vi "IMAQ_Attribute2Control_Enum.vi"(3 "error in (no error)":errorcluster, 4 "IMAQ Attribute":variant, 5 "Refnum (Enum)":refnum<vi>) -> (0 "error out":errorcluster, 1 "dup IMAQ Attribute":variant)   [LabVIEW 2012, in "HGF_VisionTools.lvlib"]
doc: "This Polymorphic VI set IMAQ control properties of type enumeration according to variant inputp value and its attribute."
uses:
  HGF_VisionTools.lvlib
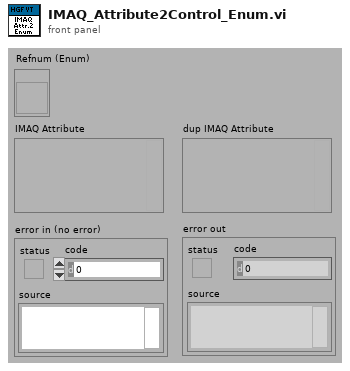
[diagram p1: front panel]
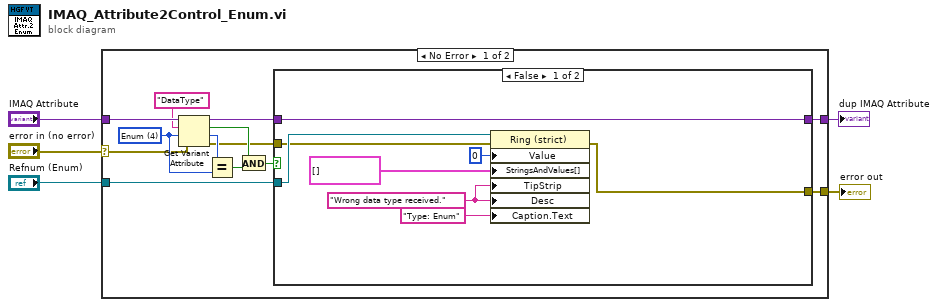
[diagram p0: block diagram]
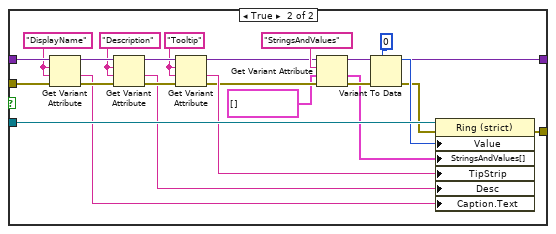
[diagram p2: hidden frame]
diagram:
  n1 = case shown="No Error" "error in (no error)" {
    selector: "error in (no error)" -> [w11 w52]
    tunnel: "IMAQ Attribute" -> [w18 w51]
    tunnel: "Refnum (Enum)" -> [w8 _]
    tunnel: [w7 w52] -> w2
    tunnel: [w6 w51] -> w1
    frame No Error {
      w15 = u32 4 items=["U32", "I64", "DBL", "String", "Enum", "Bool", "Command"] ("Type")
      n2 = Get Variant Attribute(Variant=w18, name="DataType", default value (empty Variant)=w15, error in=w11) -> (duplicate Variant=w10:variant, found=w14:bool, value=w16:u32, error out=w9:errorcluster)
      n3 = Equal?(x=w16, y=w15) -> (x = y?=w13:bool)
      n4 = And(x=w14, y=w13) -> (x .and. y?=w12:bool)
      n5 = case shown="False" w12 {
        tunnel: w10 -> [w26 w50]
        tunnel: w9 -> [w24 w49]
        tunnel: w8 -> [w25 w48]
        tunnel: [w20 w33] -> w7
        tunnel: [w26 w32] -> w6
        frame False {
          w21 = "Wrong data type received." ("Caption.Text")
          n6 = property class="Ring (strict)"(reference=w25, error in=w24, "Value"=u16 0, "StringsAndValues[]"=cluster{"String":string, "Value":u32}[] [] ("Strings And Values []"), "TipStrip"=w21, "Desc"=w21, "Caption.Text"="Type: Enum") -> (error out=w20:errorcluster)  [unwired: 1 out]
        }
        frame True {
          w38 = "Tooltip" ("name")
          w37 = "Description" ("name")
          w36 = "DisplayName" ("name")
          n7 = Get Variant Attribute(Variant=w50, name=w36, default value (empty Variant)=w36, error in=w49) -> (duplicate Variant=w45:variant, value=w34:string, error out=w46:errorcluster)  [unwired: 1 out]
          n8 = Get Variant Attribute(Variant=w45, name=w37, default value (empty Variant)=w37, error in=w46) -> (duplicate Variant=w44:variant, value=w35:string, error out=w47:errorcluster)  [unwired: 1 out]
          n9 = Get Variant Attribute(Variant=w44, name=w38, default value (empty Variant)=w38, error in=w47) -> (duplicate Variant=w31:variant, value=w39:string, error out=w30:errorcluster)  [unwired: 1 out]
          n10 = Get Variant Attribute(Variant=w31, name="StringsAndValues", default value (empty Variant)=cluster{"String":string, "Value":u32}[] [] ("Strings And Values []"), error in=w30) -> (duplicate Variant=w32:variant, value=w27:cluster{"String":string, "Value":u32}[], error out=w42:errorcluster)  [unwired: 1 out]
          n11 = Variant To Data(error in=w42, type=u32 0 ("Value"), Variant=w32) -> (data=w41:u32, error out=w40:errorcluster)
          n12 = property class="Ring (strict)"(reference=w48, error in=w40, "Value"=w41, "StringsAndValues[]"=w27, "TipStrip"=w39, "Desc"=w35, "Caption.Text"=w34) -> (error out=w33:errorcluster)  [unwired: 1 out]
        }
      }
    }
    frame Error {
    }
  }
  "error out" <- w2
  "dup IMAQ Attribute" <- w1
